vi "Check Value Type.vi"(8 "error in (no error)":errorcluster, 11 "Text Column in":refnum<class "String Column.lvclass">) -> (0 "error out":errorcluster, 3 "Text Column out":refnum<class "String Column.lvclass">)   [LabVIEW 2020, in "Basic Columns.lvlib" / "String Column.lvclass"]
uses:
  String Column.lvclass
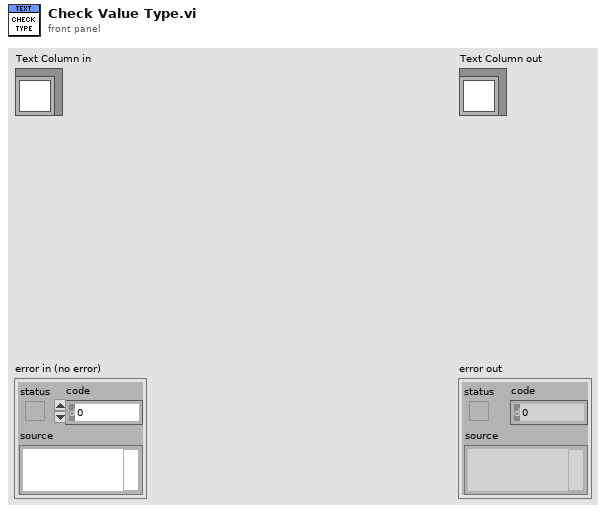
[diagram p1: front panel]
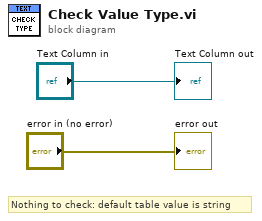
[diagram p0: block diagram]
diagram:
  # "Nothing to check: default table value is string"
  "error out" <- "error in (no error)"
  "Text Column out" <- "Text Column in"
